vi "Compute Shift.vi"(6 "chip select  (1st chip)":enum16{"1st chip", "2nd chip"}(ring), 8 "error in (no error)":errorcluster, 10 "shift direction":enum16{"left", "right"}(ring), 11 "cluster of private data in":T1={"FPGA VI Reference"=refnum, "device index"=0, "screen size"=enum."8x1", "font size"=enum."5x8", "auto wrap"=FALSE, "alignment"=enum."None", "number of line"=enum."2 lines", "shift 0"=0, "entry mode 0"=enum."increment & no shift", "shift 1"=0, "entry mode 1"=enum."increment & no shift"}) -> (0 "error out":errorcluster, 3 "cluster of private data out":T1={"FPGA VI Reference"=refnum, "device index"=0, "screen size"=enum."8x1", "font size"=enum."5x8", "auto wrap"=FALSE, "alignment"=enum."None", "number of line"=enum."2 lines", "shift 0"=0, "entry mode 0"=enum."increment & no shift", "shift 1"=0, "entry mode 1"=enum."increment & no shift"})   [LabVIEW 2017, in "HD44780.lvclass"]
uses:
  HD44780.lvclass
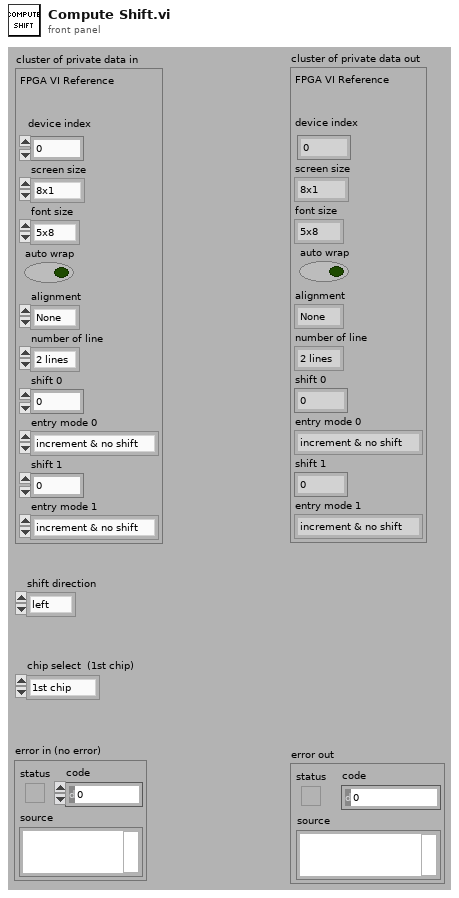
[diagram p1: front panel]
types:
  T1 = cluster{"FPGA VI Reference":refnum<k20>, "device index":i8, "screen size":enum8{"8x1", "8x2", "12x4", "16x1", "16x2", "16x4", "20x1", "20x2", "20x4", "24x1", "24x2", "40x2", "40x4"}, "font size":enum8{"5x8", "5x10"}, "auto wrap":bool, "alignment":enum16{"None", "Left", "Center", "Right"}, "number of line":enum8{"1 line", "2 lines"}, "shift 0":i8, "entry mode 0":enum8{"increment & no shift", "increment & shift", "decrement & no shift", "decrement & shift"}, "shift 1":i8, "entry mode 1":enum8{"increment & no shift", "increment & shift", "decrement & no shift", "decrement & shift"}}
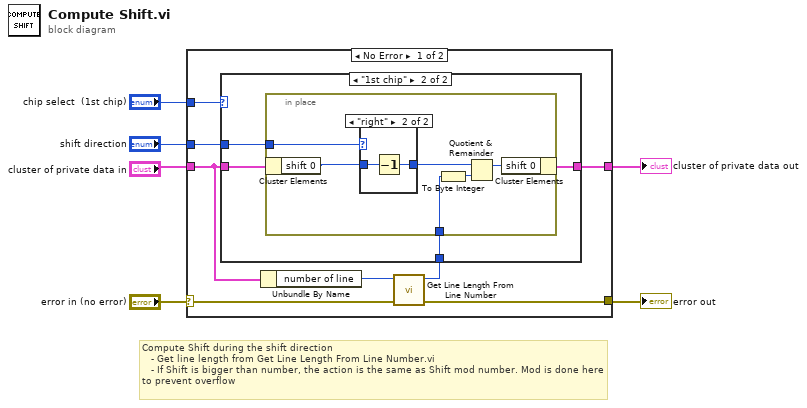
[diagram p0: block diagram]
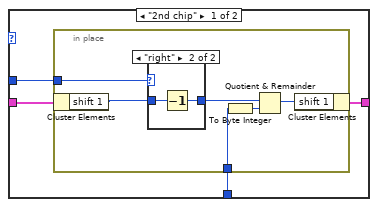
[diagram p2: hidden frame]
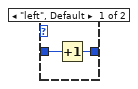
[diagram p3: hidden frame]
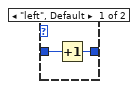
[diagram p4: hidden frame]
diagram:
  # "Compute Shift during the shift direction\n   - Get line length from Get Line Length From Line Number.vi\n   - If Shift is bigger than number, the action is the same as Shift mod number. Mod is done here to prevent overflow"
  n1 = case shown="No Error" "error in (no error)" {
    selector: "error in (no error)" -> [w8 w43]
    tunnel: "chip select  (1st chip)" -> [w12 _]
    tunnel: "shift direction" -> [w11 _]
    tunnel: [w9 w42] -> w1
    tunnel: [w8 w43] -> w3
    tunnel: "cluster of private data in" -> [w7 w42]
    frame No Error {
      n2 = Unbundle By Name(w7) -> ("number of line"=w13:enum8{"1 line", "2 lines"})
      n3 = call "Get Line Length From Line Number.vi"("line number"=w13) -> ("line length"=w10:u8)  [unwired: 10 in]
      n4 = case shown="\"1st chip\"" w12 {
        tunnel: w7 -> [w15 w29]
        tunnel: w11 -> [w17 w31]
        tunnel: w10 -> [w16 w30]
        tunnel: [w14 w28] -> w9
        frame "2nd chip" {
          n5 = in-place {
            in-place-border: w17 -> [w23]
            in-place-border: w16 -> [w18]
            n6 = in-place-cluster #1(w15) -> ("shift 1"=w22:i8)
            n7 = case shown="\"right\"" w23 {
              tunnel: w22 -> [w25 w27]
              tunnel: [w24 w26] -> w21
              frame "left", Default {
                n8 = Increment(x=w25) -> (x+1=w24:i8)
              }
              frame "right" {
                n9 = Decrement(x=w27) -> (x-1=w26:i8)
              }
            }
            n10 = To Byte Integer(number=w18) -> (8bit integer=w19:i8)
            n11 = Quotient & Remainder(x=w21, y=w19) -> (x-y*floor(x/y)=w20:i8)  [unwired: 1 out]
            n12 = in-place-cluster #1("shift 1"=w20) -> (w14:T1)
          }
        }
        frame "1st chip" {
          n13 = in-place {
            in-place-border: w31 -> [w37]
            in-place-border: w30 -> [w33]
            n14 = in-place-cluster #2(w29) -> ("shift 0"=w36:i8)
            n15 = case shown="\"right\"" w37 {
              tunnel: w36 -> [w39 w41]
              tunnel: [w38 w40] -> w35
              frame "left", Default {
                n16 = Increment(x=w39) -> (x+1=w38:i8)
              }
              frame "right" {
                n17 = Decrement(x=w41) -> (x-1=w40:i8)
              }
            }
            n18 = To Byte Integer(number=w33) -> (8bit integer=w32:i8)
            n19 = Quotient & Remainder(x=w35, y=w32) -> (x-y*floor(x/y)=w34:i8)  [unwired: 1 out]
            n20 = in-place-cluster #2("shift 0"=w34) -> (w28:T1)
          }
        }
      }
    }
    frame Error {
    }
  }
  "error out" <- w3
  "cluster of private data out" <- w1
